vi "Discovery Connection Manager Loop.vi"(0 "stop notifier":refnum<notifier>, 5 "discovered host queue":refnum<queue>, 7 "Discovery Events":T1, 9 "stale threshold (s)":dbl=5.0) -> (15 "error out":errorcluster)   [LabVIEW 2020, in "epl-network.lvlib"]
uses:
  epl-network.lvlib
  Discovery Events.ctl
  Public/Discovery/Typedefs/Server Beacon.ctl
  Discovered Host.ctl
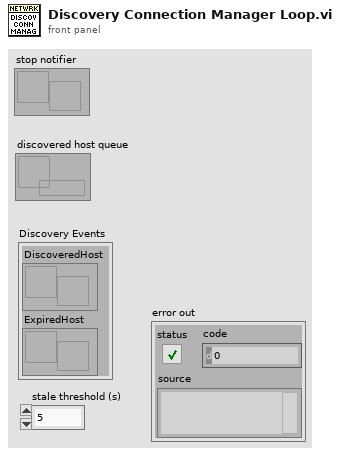
[diagram p1: front panel]
types:
  T1 = typedef "epl-network.lvlib/Discovery Events.ctl" = cluster{"DiscoveredHost":refnum<user-event>, "ExpiredHost":refnum<user-event>}
  T2 = typedef "epl-network.lvlib/Discovered Host.ctl" = cluster{"Beacon":T3, "Last Seen":timestamp}
  T3 = typedef "epl-network.lvlib/Server Beacon.ctl" = cluster{"name":string, "addr":string, "port":u16, "ver":u16}
  T4 = typedef "epl-network.lvlib/Beacon Result.ctl" = enum16{"Ignored", "Updated", "Added"}
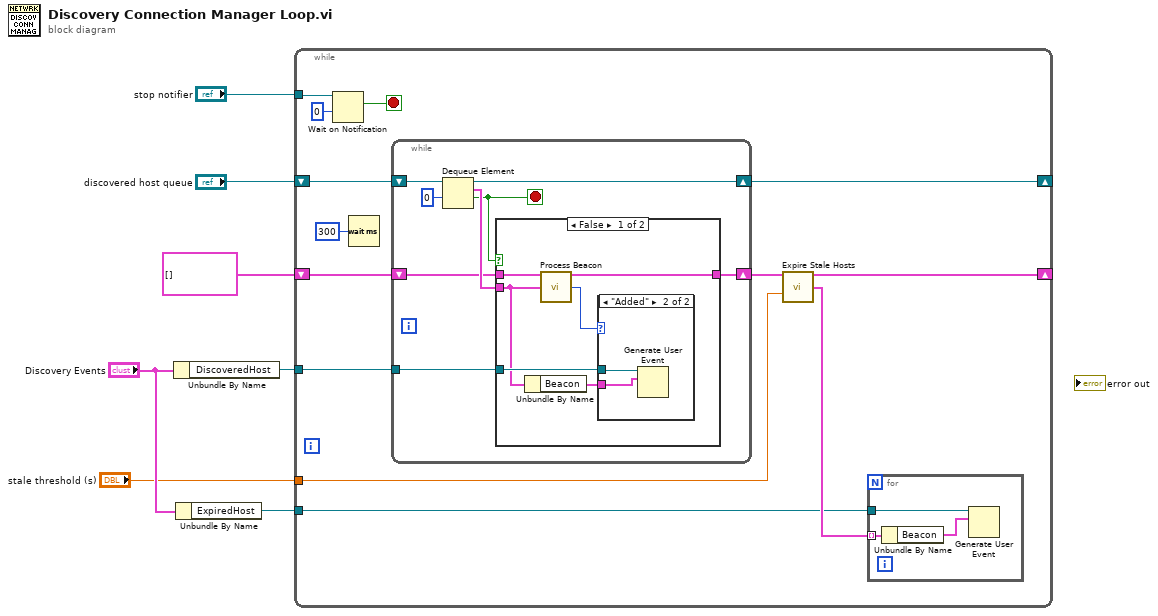
[diagram p0: block diagram]
diagram:
  n1 = Unbundle By Name("Discovery Events") -> ("DiscoveredHost"=w6:refnum<user-event>)
  n2 = Unbundle By Name("Discovery Events") -> ("ExpiredHost"=w2:refnum<user-event>)
  n3 = while {
    shift-right: [w18] -> _
    shift-left: "discovered host queue" -> [w20]
    shift-right: [w11] -> _
    shift-left: T2[] [] ("Array") -> [w19]
    tunnel: w6 -> [w17]
    tunnel: "stop notifier" -> [w14]
    tunnel: w2 -> [w9]
    tunnel: "stale threshold (s)" -> [w8]
    stop <- w13 stop-if-true
    n4 = Wait on Notification(notifier=w14, timeout in ms (-1)=0) -> (notification=w13:bool)  [unwired: 2 in, 3 out]
    n5 = Wait (ms)(milliseconds to wait=u32 300) -> ()  [unwired: 1 out]
    n6 = while {
      shift-right: [w29] -> w18
      shift-left: w20 -> [w31]
      shift-right: [w28] -> w12
      shift-left: w19 -> [w24]
      tunnel: w17 -> [w27]
      stop <- w25 stop-if-true
      n7 = Dequeue Element(queue=w31, timeout in ms (-1)=0) -> (queue out=w29:refnum<queue>, element=w26:T2, timed out?=w25:bool)  [unwired: 1 in, 1 out]
      n8 = case shown="False" w25 {
        tunnel: [w37 w40] -> w28
        tunnel: w27 -> [w35 _]
        tunnel: w26 -> [w34 _]
        tunnel: w24 -> [w32 w40]
        frame False {
          n9 = Unbundle By Name(w34) -> ("Beacon"=w33:T3)
          n10 = call "Process Beacon.vi"("Known Hosts in"=w32, "DiscoveredHost"=w34) -> ("Known Hosts out"=w37:T2[], "Beacon Result"=w36:T4)  [unwired: 12 in]
          n11 = case shown="\"Added\"" w36 {
            tunnel: w35 -> [_ w39]
            tunnel: w33 -> [_ w38]
            frame "Ignored", Default {
            }
            frame "Added" {
              n12 = Generate User Event(user event=w39, event data cluster=w38) -> ()  [unwired: 2 in, 2 out]
            }
          }
        }
        frame True {
        }
      }
    }
    n13 = call "Expire Stale Hosts.vi"("Known Hosts in"=w12, "timeout (s)"=w8) -> ("Known hosts out"=w11:T2[], "Expired"=w10:T2[])  [unwired: 12 in]
    n14 = for {
      tunnel: w10 -> [w22] mode=indexing
      tunnel: w9 -> [w23]
      n15 = Unbundle By Name(w22) -> ("Beacon"=w21:T3)
      n16 = Generate User Event(user event=w23, event data cluster=w21) -> ()  [unwired: 2 in, 2 out]
    }
  }
